vi "DataTranslation.vi"() -> (0 "DAQ Error":errorcluster)   [LabVIEW 2017]
doc: "This vi will take data with multiple DT boxes for an arbitrary number of channels either differentially or single ended, depending upon how you have wired the boxes up."
uses:
  Controls/DT_Cluster.ctl
  Controls/DT_Mode.ctl
  Globals/Meas_global.vi
  <userlib>/LV-Link3/PolySubVIs/DtOLReadMultiple2D.vi
  <userlib>/LV-Link3/PolySubVIs/DtOLTriggerDigital.vi
  <userlib>/LV-Link3/PolySubVIs/DtOLStartNormal.vi
  <userlib>/LV-Link3/PolySubVIs/DtOLTimingSetInput.vi
  <userlib>/LV-Link3/PolySubVIs/DtCreateCtrRateChan.vi
  <userlib>/LV-Link3/PolySubVIs/DtCreateAinChan.vi
  Globals/Trav_pos_global.vi
  Globals/Extra_Commands_Global.vi
  Globals/Dynamic_call_global.ph.vi
panel:
  out "Array":T1[](array[typedef])
  out "Waveform Graph":dbl[][](graph)
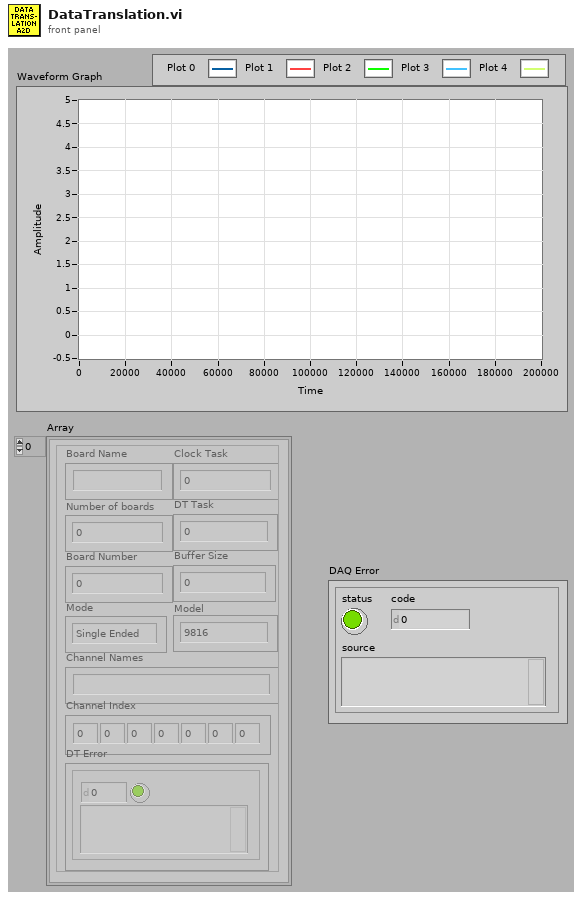
[diagram p1: front panel]
types:
  T1 = typedef "DT_Cluster.ctl" = cluster{"Board Name":string, "Number of boards":u32, "Board Number":u32, "Channel Names":string, "Channel Index":i32[], "DT Task":i32, "DT Error":errorcluster, "Mode":T2, "Buffer Size":u32, "Clock Task":i32, "Model":enum16{"9816", "9836", "9853"}}
  T2 = typedef "DT_Mode.ctl" = enum16{"Single Ended", "Differential"}
  T3 = typedef "Trigger_Mode.ctl" = enum16{"Free Running", "Start on Trigger", "Trigger Every Block", "Trigger Every Sample"}
  T4 = typedef "LDA_Setup.ctl" = cluster{"dimensions":enum16{"1D", "2D"}, "Analogue Freq Multiplier":dbl}
  T5 = enum32{"Internal Clock", "External Clock", "No Timing"}
  T6 = typedef "Traverse_cluster.ctl" = cluster{"Start X":sgl, "Start Y":sgl, "Start Z":sgl, "End X":sgl, "End Y":sgl, "End Z":sgl, "No. of pts.":i32, "Spacing":T7, "Filename":path, "Tunnel Speed":dbl, "Averaging time (min)":dbl, "Extra Commands":string, "Carrier_1 Q (l/min)":dbl, "Carrier_2 Q (l/min)":dbl, "Trace Gas Concentration (%)":dbl, "Specific Arguments":string, "Comments":string, "Row No":i32, "Row Type Selector":T8, "Completion time":string, "Row Duration (mins)":dbl, "No. of Valid pts.":i32, "Meas Setup File":string}
  T7 = typedef "Spacing.ctl" = enum16{"Linear", "Log", "Gauss", "Specified", "N/A"}
  T8 = typedef "Multi_run_mode.ctl" = enum16{"Move Traverse Only", "Set Tunnel Speed Only", "Set Source Only", "Set Measurement Conditions", "Single Measurement", "Vertical Profile", "Lateral Profile", "Longitudinal Profile", "Explore Volume", "Multi-Axis Profile", "Auto Calibrate", "Meas Fast FID Bkgnd", "Check Beam Power", "Scanning Valve Measurement", "Run VI Named:", "Set ADAM Ch", "Wait (minutes)", "Send Message", "Synchronize With:", "Fall Back to this Row", "Turn Off Row Repeating", "Blank Row", "Traverse 3D Volume"}
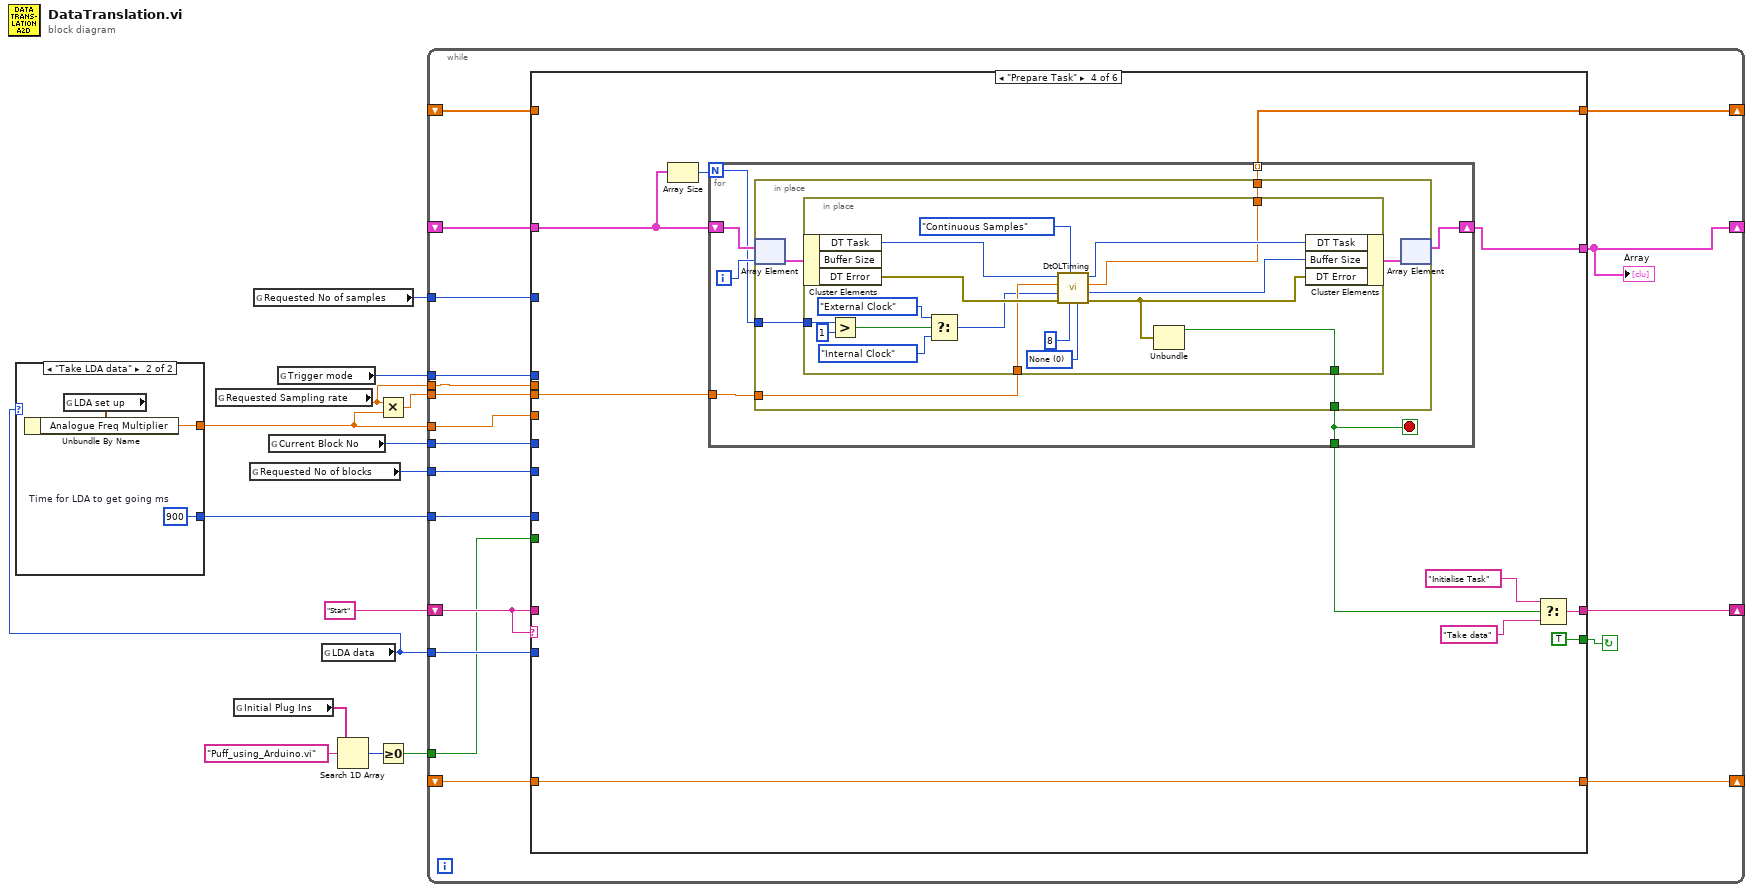
[diagram p0: block diagram]
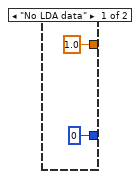
[diagram p2: hidden frame]
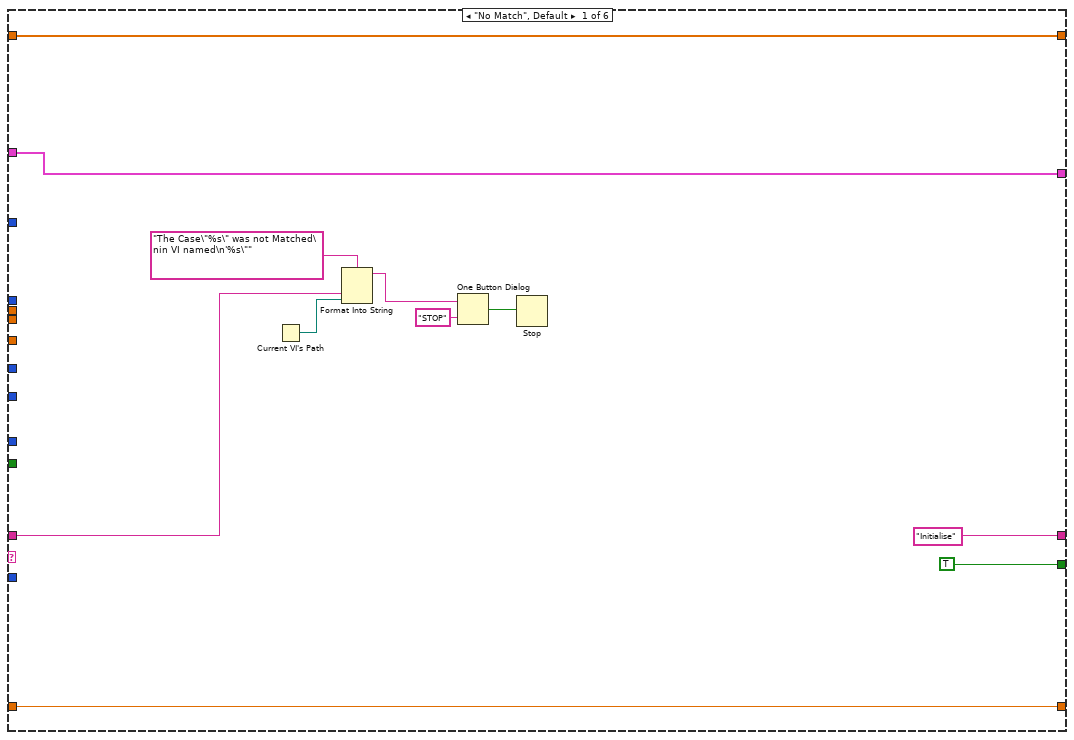
[diagram p3: hidden frame]
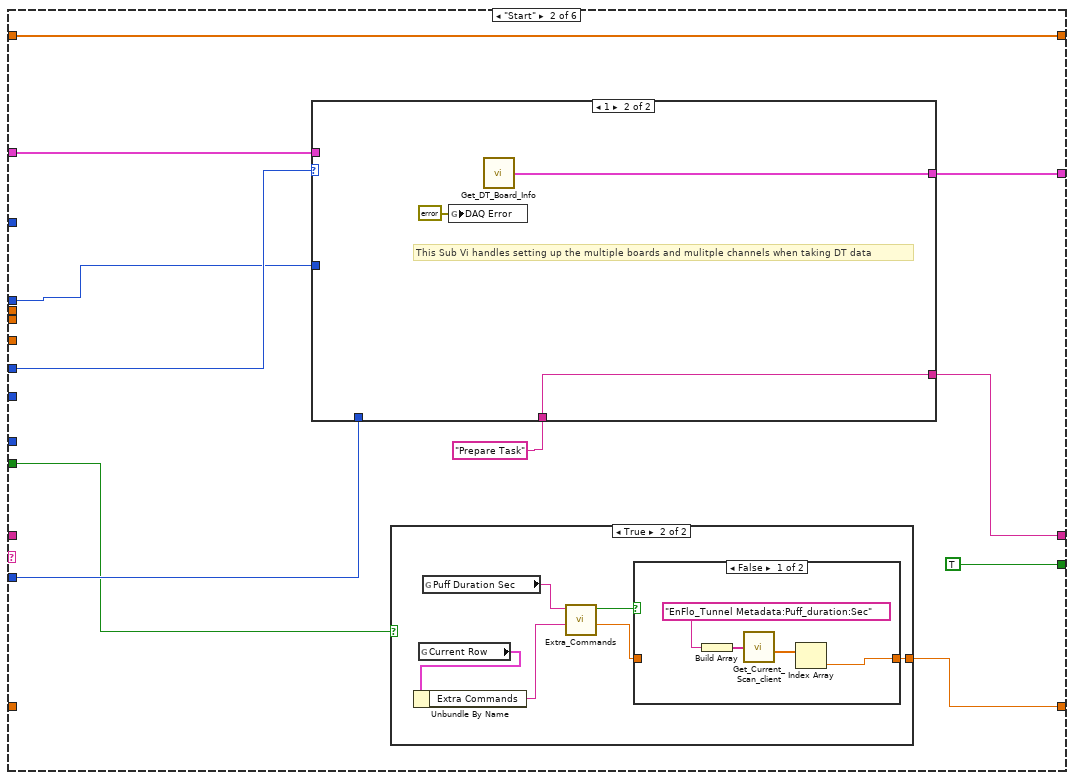
[diagram p4: hidden frame]
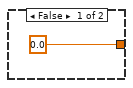
[diagram p5: hidden frame]
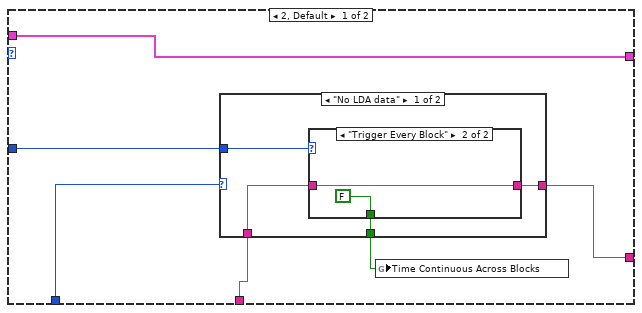
[diagram p7: hidden frame]
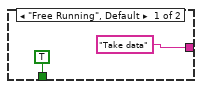
[diagram p8: hidden frame]
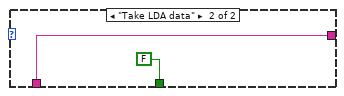
[diagram p9: hidden frame]
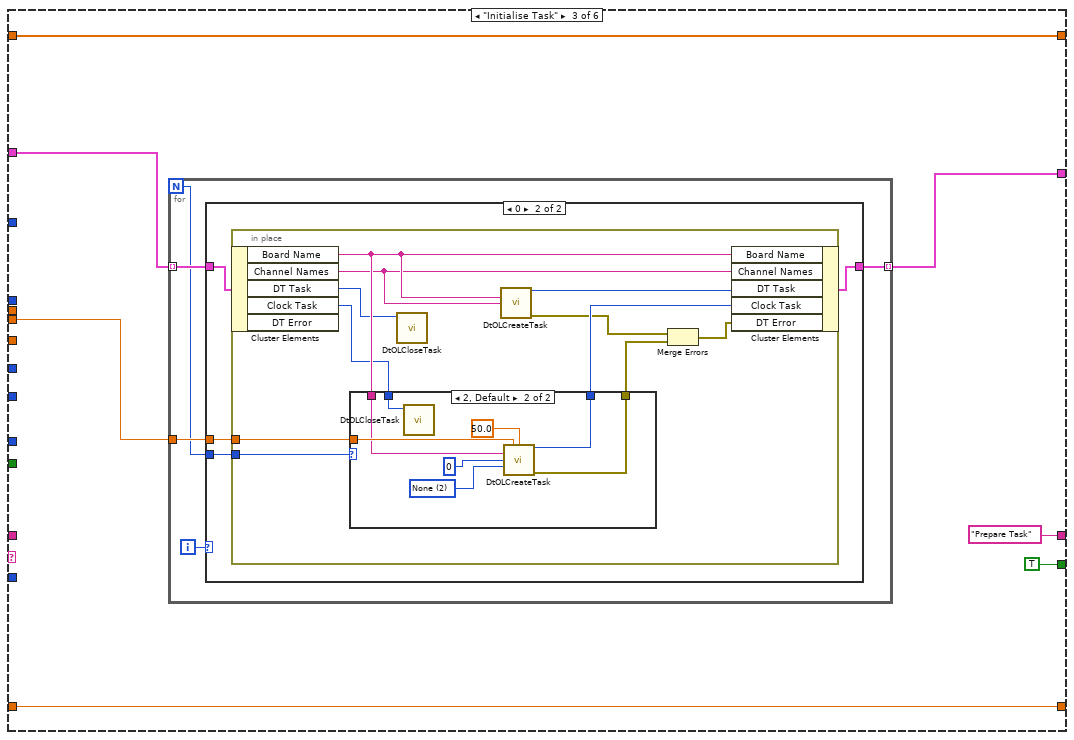
[diagram p10: hidden frame]
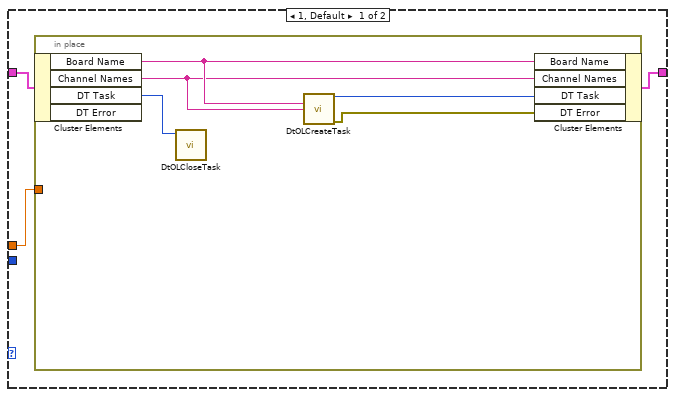
[diagram p11: hidden frame]
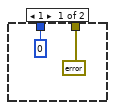
[diagram p12: hidden frame]
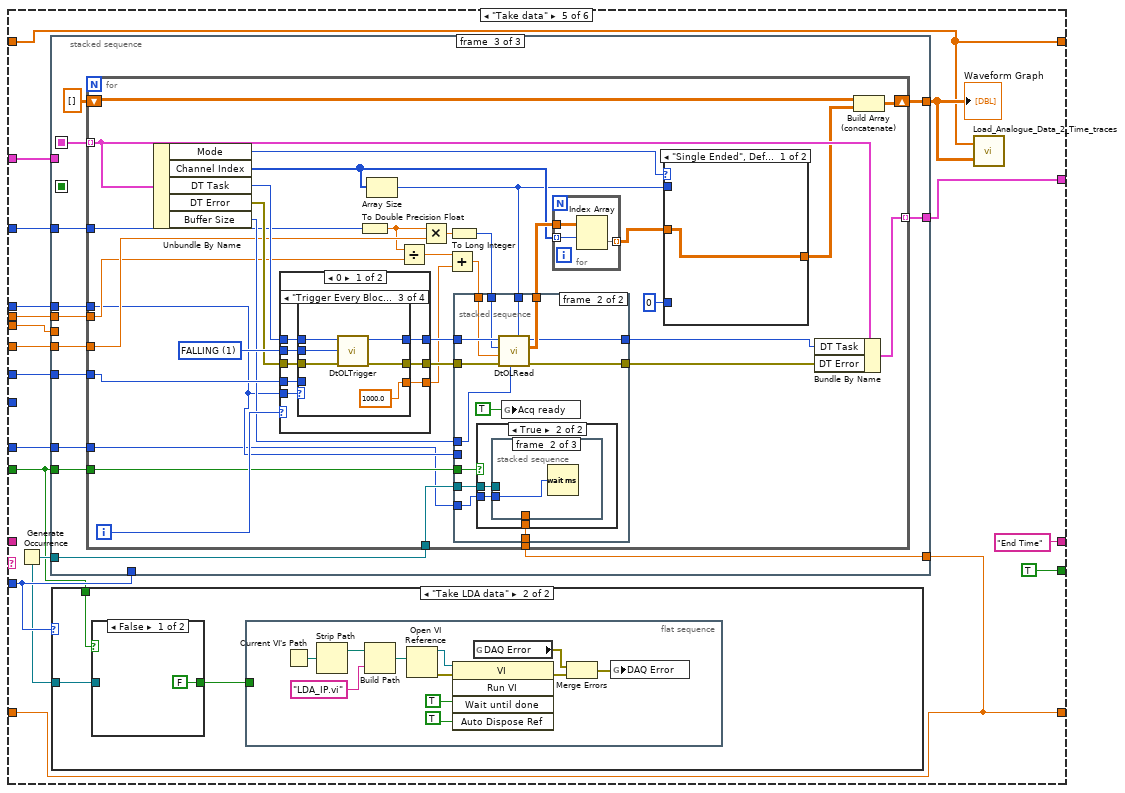
[diagram p13: hidden frame]
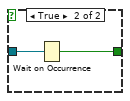
[diagram p15: hidden frame]
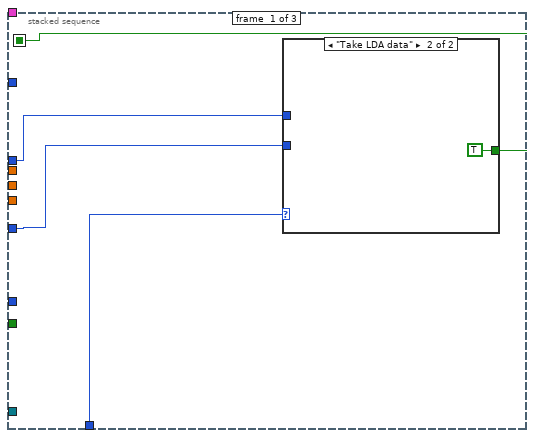
[diagram p16: hidden frame]
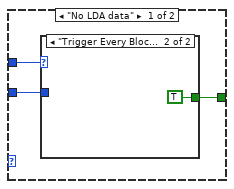
[diagram p17: hidden frame]
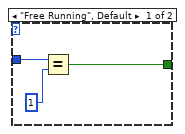
[diagram p18: hidden frame]
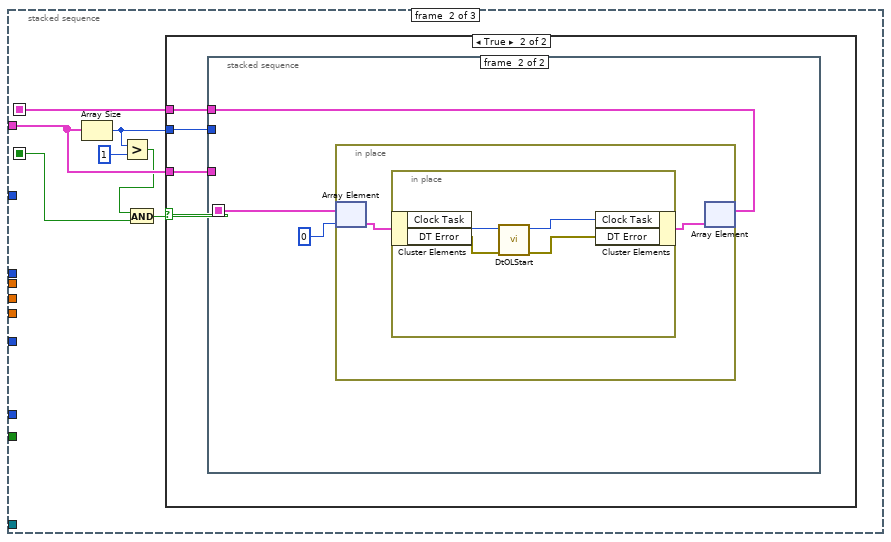
[diagram p19: hidden frame]
diagram:
  n1 = global read "Meas_global.vi" "Requested Sampling rate"() -> (w9:dbl)
  n2 = global read "Dynamic_call_global.ph.vi" "Initial Plug Ins"() -> (w5:string[])
  n3 = global read "Meas_global.vi" "Requested No of blocks"() -> (w8:i32)
  n4 = global read "Meas_global.vi" "Requested No of samples"() -> (w13:i32)
  n5 = global read "Meas_global.vi" "Current Block No"() -> (w11:i32)
  n6 = global read "Meas_global.vi" "Trigger mode"() -> (w12:T3)
  n7 = global read "Meas_global.vi" "LDA data"() -> (w6:enum16{"No LDA data", "Take LDA data"})
  n8 = case shown="\"Take LDA data\"" w6 {
    tunnel: [1.0 ("Analogue Freq Multiplier") w18] -> w7
    tunnel: [u32 0 ("Time for LDA to get going ms") w17] -> w1
    frame "No LDA data" {
    }
    frame "Take LDA data" {
      w17 = u32 900  # Time for LDA to get going ms
      n9 = global read "Meas_global.vi" "LDA set up"() -> (w19:T4)
      n10 = Unbundle By Name(w19) -> ("Analogue Freq Multiplier"=w18:dbl)
    }
  }
  n11 = Search 1D Array(1D array=w5, element="Puff_using_Arduino.vi") -> (index of element=w3:i32)  [unwired: 1 in]
  n12 = Multiply(x=w9, y=w7) -> (x*y=w10:dbl)
  n13 = Greater Or Equal To 0?(x=w3) -> (x >= 0?=w2:bool)
  n14 = while {
    shift-left: "Start" -> [w37]
    shift-right: [w38] -> _
    tunnel: w10 -> [w36]
    tunnel: w13 -> [w35]
    tunnel: w11 -> [w34]
    tunnel: w12 -> [w32]
    shift-right: [w31] -> _
    shift-left: _ -> [w30]
    tunnel: w6 -> [w29]
    tunnel: w7 -> [w28]
    tunnel: w9 -> [w27]
    tunnel: w8 -> [w26]
    tunnel: w2 -> [w25]
    shift-right: [w24] -> _
    shift-left: _ -> [w23]
    tunnel: w1 -> [w22]
    shift-right: [w21] -> _
    shift-left: _ -> [w20]
    stop <- w33 continue-if-true
    n15 = case shown="\"Prepare Task\"" w37 {
      tunnel: ["Initialise" w56 "Prepare Task" w144 "End Time" "" ("f")] -> w38
      tunnel: w37 -> [w45 _ _ _ _ _]
      tunnel: w36 -> [_ _ w96 w140 w185 _]
      tunnel: w35 -> [_ _ _ _ w193 _]
      tunnel: w34 -> [_ w57 _ _ w191 w386]
      tunnel: [TRUE TRUE TRUE TRUE TRUE FALSE] -> w33
      tunnel: w32 -> [_ w53 _ _ w190 _]
      tunnel: w30 -> [w41 w58 w94 w139 w189 w390]
      tunnel: [w41 w59 w95 w141 w188 w389] -> w31
      tunnel: w29 -> [_ w54 _ _ w184 _]
      tunnel: w28 -> [_ _ _ _ w187 _]
      tunnel: w27 -> [_ _ _ _ w186 _]
      tunnel: w26 -> [_ _ _ _ _ w387]
      tunnel: w25 -> [_ w52 _ _ w181 _]
      tunnel: [w40 w51 w93 w138 w182 w382] -> w24
      tunnel: w23 -> [w40 _ w93 w138 w182 w382]
      tunnel: w22 -> [_ _ _ _ w180 _]
      tunnel: [w39 w50 w92 w137 w178 w381] -> w21
      tunnel: w20 -> [w39 w50 w92 _ w178 w381]
      frame "No Match", Default {
        n16 = Current VI's Path() -> (path=w44:path)
        n17 = Format Into String(format string="The Case\"%s\" was not Matched\nin VI named\n'%s\"" ("Format String"), w45, w44) -> (resulting string=w48:string)  [unwired: 2 in, 1 out]
        n18 = One Button Dialog(message=w48, button name ("OK")="STOP") -> (true=w46:bool)
        n19 = Stop(stop? (T)=w46) -> ()
      }
      frame "Start" {
        n20 = case shown="1" w57 {
          tunnel: [w78 w91] -> w59
          tunnel: w58 -> [w78 _]
          tunnel: [w76 w89] -> w56
          tunnel: "Prepare Task" -> [w75 w89]
          tunnel: w54 -> [w77 _]
          tunnel: w53 -> [w74 _]
          frame 2, Default {
            n21 = case shown="\"No LDA data\"" w77 {
              tunnel: [w82 w88] -> w76
              tunnel: w75 -> [w80 w88]
              tunnel: w74 -> [w81 _]
              tunnel: [w79 FALSE ("Time Continuous across Blocks")] -> w73
              frame "No LDA data" {
                n22 = case shown="\"Trigger Every Block\"" w81 {
                  tunnel: ["Take data" w86] -> w82
                  tunnel: w80 -> [_ w86]
                  tunnel: [TRUE ("Time Continuous across Blocks") FALSE ("Time Continuous across Blocks")] -> w79
                  frame "Free Running", Default {
                  }
                  frame "Trigger Every Block" {
                  }
                }
              }
              frame "Take LDA data" {
              }
            }
            n23 = global write "Meas_global.vi" "Time Continuous Across Blocks"(w73) -> ()
          }
          frame 1 {
            # "This Sub Vi handles setting up the multiple boards and mulitple channels when taking DT data"
            n24 = global write "Meas_global.vi" "DAQ Error"(errorcluster {"status"=FALSE, "code"=0, "source"=""} ("DAQ Error")) -> ()
            n25 = call "Get_DT_Board_Info.vi"() -> ("DT Cluster Array"=w91:T1[])  [unwired: 5 in]
          }
        }
        n26 = case shown="True" w52 {
          tunnel: [0.0 w67] -> w51
          frame False {
          }
          frame True {
            n27 = global read "Trav_pos_global.vi" "Current Row"() -> (w66:T6)
            n28 = Unbundle By Name(w66) -> ("Extra Commands"=w65:string)
            n29 = global read "Extra_Commands_Global.vi" "Puff Duration Sec"() -> (w64:string)
            n30 = call "Extra_Commands.vi"("String to Search"=w65, "Command"=w64) -> ("Numeric Value"=w62:dbl, "Command Found"=w63:bool)  [unwired: 2 in, 2 out]
            n31 = case shown="False" w63 {
              tunnel: [w68 w72] -> w67
              tunnel: w62 -> [_ w72]
              frame False {
                n32 = Build Array("EnFlo_Tunnel Metadata:Puff_duration:Sec") -> (w70:string[])
                n33 = call "Get_Current_Scan_client.vi"("ADAM Ch Names"=w70) -> ("Numerical Values"=w71:dbl[])  [unwired: 1 in, 2 out]
                n34 = Index Array(array=w71) -> (element=w68:dbl)  [unwired: 1 in]
              }
              frame True {
              }
            }
          }
        }
      }
      frame "Initialise Task" {
        n35 = for {
          N -> [w99]
          tunnel: w94 -> [w103] mode=indexing
          tunnel: w96 -> [w102]
          tunnel: [w101] -> w95 mode=indexing
          i -> [w100]
          n36 = case shown="0" w100 {
            tunnel: w103 -> [w106 w115]
            tunnel: w102 -> [w105 w114]
            tunnel: [w104 w113] -> w101
            tunnel: w99 -> [_ w112]
            frame 1, Default {
              n37 = in-place {
                in-place-border: w105 -> [_]
                n38 = in-place-cluster #1(w106) -> ("Board Name"=w111:string, "Channel Names"=w108:string, "DT Task"=w107:i32)  [unwired: 1 out]
                n39 = call <userlib>:"DtOLCloseTask.vi"("Task in"=w107) -> ()  [unwired: 10 in, 1 out]
                n40 = call-poly <userlib>:"DtOLCreateTask.vi"("Board Name"=w111, "Channel"=w108) -> ("Task out"=w110:i32, "error out"=w109:errorcluster)  [unwired: 11 in, 1 out]
                n41 = in-place-cluster #1("Board Name"=w111, "Channel Names"=w108, "DT Task"=w110, "DT Error"=w109) -> (w104:T1)
              }
            }
            frame 0 {
              n42 = in-place {
                in-place-border: w114 -> [w126]
                in-place-border: w112 -> [w117]
                n43 = in-place-cluster #2(w115) -> ("Board Name"=w124:string, "Channel Names"=w119:string, "DT Task"=w118:i32, "Clock Task"=w116:i32)  [unwired: 1 out]
                n44 = case shown="2, Default" w117 {
                  tunnel: w126 -> [_ w133]
                  tunnel: [errorcluster {"status"=FALSE, "code"=0, "source"=""} ("error out") w132] -> w125
                  tunnel: w124 -> [_ w131]
                  tunnel: [0 ("Task out") w130] -> w122
                  tunnel: w116 -> [_ w129]
                  frame 1 {
                  }
                  frame 2, Default {
                    w136 = 2 items=["LowLevel", "HighLevel", "None"] ("Gate Type")
                    n45 = call <userlib>:"DtOLCloseTask.vi"("Task in"=w129) -> ()  [unwired: 10 in, 1 out]
                    n46 = call-poly <userlib>:"DtOLCreateTask.vi"("Requested\nFrequency (Hz)"=w133, "Duty Cycle"=50.0, "Board Name"=w131, "Counter Num"=u32 0, "Gate Type"=w136) -> ("Task out"=w130:i32, "error out"=w132:errorcluster)  [unwired: 8 in, 1 out]
                  }
                }
                n47 = call <userlib>:"DtOLCloseTask.vi"("Task in"=w118) -> ()  [unwired: 10 in, 1 out]
                n48 = call-poly <userlib>:"DtOLCreateTask.vi"("Board Name"=w124, "Channel"=w119) -> ("Task out"=w123:i32, "error out"=w121:errorcluster)  [unwired: 11 in, 1 out]
                n49 = Merge Errors(w121, w125) -> (w120:errorcluster)
                n50 = in-place-cluster #2("Board Name"=w124, "Channel Names"=w119, "DT Task"=w123, "Clock Task"=w122, "DT Error"=w120) -> (w113:T1)
              }
            }
          }
        }
      }
      frame "Prepare Task" {
        n51 = Array Size(array=w139) -> (size(s)=w143:i32)
        n52 = for {
          N: w143 -> [w149]
          shift-right: [w151] -> w141
          shift-left: w139 -> [w153]
          tunnel: [w154] -> w142
          tunnel: w140 -> [w150]
          tunnel: [w148] -> w137 mode=indexing
          i -> [w152]
          stop <- w154 stop-if-true
          n53 = in-place {
            in-place-border: [w160] -> w154
            in-place-border: w150 -> [w157]
            in-place-border: w149 -> [w156]
            in-place-border: [w155] -> w148
            n54 = in-place-array #3(w153, w152) -> (w159:T1)
            n55 = in-place {
              in-place-border: [w172] -> w160
              in-place-border: w157 -> [w171]
              in-place-border: w156 -> [w170]
              in-place-border: [w161] -> w155
              w163 = 0 items=["None", "Master", "Slave"] ("Sync Mode")
              n56 = in-place-cluster #4(w159) -> ("DT Task"=w177:i32, "DT Error"=w176:errorcluster)  [unwired: 1 out]
              n57 = Greater?(x=w170, y=1) -> (0:w168:bool)
              n58 = Select(t=T5."External Clock" ("Timing"), s=w168, f=T5."Internal Clock" ("Timing")) -> (s? t:f=w165:T5)
              n59 = call-poly <userlib>:"DtOLTiming.vi"("Sync Mode"=w163, "Num Buffers"=u32 8, "Sample Mode"=enum16{"Finite Samples", "Continuous Samples"}."Continuous Samples", "error in (no error)"=w176, "Timing"=w165, "Sample Freq (Hz)"=w171, "Task in"=w177) -> ("error out"=w173:errorcluster, "Buffer Size"=w175:u32, "Actual Sample Freq"=w161:dbl, "Task out"=w174:i32)  [unwired: 1 in]
              n60 = Unbundle(w173) -> ("status"=w172:bool)  [unwired: 2 out]
              n61 = in-place-cluster #4("DT Task"=w174, "Buffer Size"=w175, "DT Error"=w173) -> (w158:T1)
            }
            n62 = in-place-array #3(w158) -> (w151:T1[])  [unwired: 1 out]
          }
        }
        n63 = Select(t="Initialise Task", s=w142, f="Take data") -> (s? t:f=w144:string)
      }
      frame "Take data" {
        n64 = Generate Occurrence() -> (w183:refnum<k4>)
        n65 = stacked-sequence {
          seq-local: [_ w230 _] -> [_ _ w260]
          seq-local: [w213 _ _] -> [_ w225 _]
          tunnel: w193 -> [_ _ w268]
          tunnel: w191 -> [w214 _ w267]
          tunnel: w190 -> [w212 _ w266]
          tunnel: w189 -> [_ w229 _]
          tunnel: [_ _ w265] -> w188
          tunnel: [_ _ w263] -> w179
          tunnel: w187 -> [_ _ w262]
          tunnel: w186 -> [_ _ w261]
          tunnel: w184 -> [w215 _ _]
          tunnel: w185 -> [_ _ _]
          tunnel: w183 -> [_ _ w259]
          tunnel: w181 -> [_ _ w258]
          tunnel: w182 -> [_ _ w257]
          tunnel: w180 -> [_ _ w256]
          frame #0 {
            n66 = case shown="\"Take LDA data\"" w215 {
              tunnel: w214 -> [w218 _]
              tunnel: [w217 TRUE] -> w213
              tunnel: w212 -> [w216 _]
              frame "No LDA data" {
                n67 = case shown="\"Trigger Every Block\"" w216 {
                  tunnel: w218 -> [w221 _]
                  tunnel: [w219 TRUE] -> w217
                  frame "Free Running", Default {
                    n68 = Equal?(x=w221, y=1) -> (x = y?=w219:bool)
                  }
                  frame "Trigger Every Block" {
                  }
                }
              }
              frame "Take LDA data" {
              }
            }
          }
          frame #1 {
            n69 = Array Size(array=w229) -> (size(s)=w228:i32)
            n70 = Greater?(x=w228, y=1) -> (0:w226:bool)
            n71 = And(x=w226, y=w225) -> (x .and. y?=w224:bool)
            n72 = case shown="True" w224 {
              tunnel: [w231 w234] -> w230
              tunnel: w229 -> [w231 w233]
              tunnel: w228 -> [_ w232]
              frame False {
              }
              frame True {
                n73 = stacked-sequence {
                  seq-local: [w235 _] -> [_ w248]
                  tunnel: [_ w247] -> w234
                  tunnel: w233 -> [w237 _]
                  tunnel: w232 -> [w236 _]
                  frame #0 {
                    n74 = for {
                      N: w236 -> [_]
                      shift-right: [w238] -> w235
                      shift-left: w237 -> [w239]
                      i -> [w240]
                      n75 = in-place {
                        n76 = in-place-array #5(w239, w240) -> (w242:T1)
                        n77 = in-place {
                          n78 = in-place-cluster #6(w242) -> ("DT Task"=w246:i32, "DT Error"=w245:errorcluster)
                          n79 = call-poly <userlib>:"DtOLStart.vi"("error in (no error)"=w245, "Task in"=w246) -> ("error out"=w244:errorcluster, "Task out"=w243:i32)  [unwired: 8 in]
                          n80 = in-place-cluster #6("DT Task"=w243, "DT Error"=w244) -> (w241:T1)
                        }
                        n81 = in-place-array #5(w241) -> (w238:T1[])  [unwired: 1 out]
                      }
                    }
                  }
                  frame #1 {
                    n82 = in-place {
                      n83 = in-place-array #7(w248, 0) -> (w251:T1)
                      n84 = in-place {
                        n85 = in-place-cluster #8(w251) -> ("Clock Task"=w254:i32, "DT Error"=w255:errorcluster)
                        n86 = call-poly <userlib>:"DtOLStart.vi"("error in (no error)"=w255, "Task in"=w254) -> ("error out"=w252:errorcluster, "Task out"=w253:i32)  [unwired: 8 in]
                        n87 = in-place-cluster #8("Clock Task"=w253, "DT Error"=w252) -> (w250:T1)
                      }
                      n88 = in-place-array #7(w250) -> (w247:T1[])  [unwired: 1 out]
                    }
                  }
                }
              }
            }
          }
          frame #2 {
            n89 = for {
              tunnel: w268 -> [w283]
              tunnel: w267 -> [w301]
              tunnel: w266 -> [w270]
              tunnel: w260 -> [w297] mode=indexing
              tunnel: [w296] -> w265 mode=indexing
              shift-right: [w293] -> w263
              shift-left: dbl[][] [] -> [w292]
              tunnel: w262 -> [w282]
              tunnel: w261 -> [w280]
              tunnel: w259 -> [w273]
              tunnel: w258 -> [w272]
              tunnel: w257 -> [w271]
              tunnel: w256 -> [w269]
              i -> [w290]
              w302 = 1 items=["RISING", "FALLING"] ("External Trigger Polarity")
              n90 = Unbundle By Name(w297) -> ("Mode"=w287:T2, "Channel Index"=w294:i32[], "DT Task"=w300:i32, "DT Error"=w299:errorcluster, "Buffer Size"=w285:u32)
              n91 = case shown="0" w290 {
                tunnel: [w346 w377] -> w303
                tunnel: w302 -> [w345 _]
                tunnel: w301 -> [w344 _]
                tunnel: w270 -> [w343 _]
                tunnel: w300 -> [w342 w377]
                tunnel: w299 -> [w341 w376]
                tunnel: [w340 w376] -> w298
                tunnel: [w339 10.0 ("x")] -> w277
                frame 0 {
                  n92 = case shown="\"Trigger Every Block\"" w343 {
                    tunnel: [w349 w354 w369 w374] -> w346
                    tunnel: w342 -> [w349 w355 w371 w374]
                    tunnel: w344 -> [_ w356 _ _]
                    tunnel: w345 -> [_ w353 w370 _]
                    tunnel: w341 -> [w348 w352 w368 w373]
                    tunnel: [w348 w351 w367 w373] -> w340
                    tunnel: [10.0 ("x") w350 1000.0 ("x") 1000.0 ("x")] -> w339
                    frame "Free Running" {
                    }
                    frame "Start on Trigger" {
                      n93 = case shown="1" w356 {
                        tunnel: w355 -> [w362 w365]
                        tunnel: w352 -> [w361 w364]
                        tunnel: [w359 w365] -> w354
                        tunnel: [w360 w364] -> w351
                        tunnel: w353 -> [w358 _]
                        tunnel: [1000.0 ("x") 10.0 ("x")] -> w350
                        frame 1 {
                          n94 = call-poly <userlib>:"DtOLTrigger.vi"("error in (no error)"=w361, "External Trigger Polarity"=w358, "Task in"=w362) -> ("error out"=w360:errorcluster, "Task out"=w359:i32)  [unwired: 7 in]
                        }
                        frame 2, Default {
                        }
                      }
                    }
                    frame "Trigger Every Block" {
                      n95 = call-poly <userlib>:"DtOLTrigger.vi"("error in (no error)"=w368, "External Trigger Polarity"=w370, "Task in"=w371) -> ("error out"=w367:errorcluster, "Task out"=w369:i32)  [unwired: 7 in]
                    }
                    frame "Trigger Every Sample" {
                    }
                  }
                }
                frame 1, Default {
                }
              }
              n96 = To Double Precision Float(number=w283) -> (double precision float=w275:dbl)
              n97 = Array Size(array=w294) -> (size(s)=w276:i32)
              n98 = Divide(x=w275, y=w280) -> (x/y=w278:dbl)
              n99 = Multiply(x=w275, y=w282) -> (x*y=w281:dbl)
              n100 = Add(x=w278, y=w277) -> (x+y=w291:dbl)
              n101 = To Long Integer(number=w281) -> (32bit integer=w274:i32)
              n102 = stacked-sequence {
                tunnel: w303 -> [_ w320]
                tunnel: w298 -> [_ w319]
                tunnel: [_ w318] -> w295
                tunnel: w291 -> [_ w317]
                tunnel: [_ w316] -> w289
                tunnel: w285 -> [_ w312]
                tunnel: [_ w315] -> w284
                tunnel: w274 -> [_ w314]
                tunnel: w276 -> [_ w313]
                tunnel: w273 -> [_ w310]
                tunnel: w272 -> [_ w309]
                tunnel: w271 -> [_ w308]
                tunnel: w270 -> [w305 _]
                tunnel: w269 -> [w304 w307]
                frame #0 {
                  n103 = case shown="\"Free Running\"" w305 {
                    tunnel: w304 -> [w306 _]
                    frame "Free Running" {
                      n104 = Wait (ms)(milliseconds to wait=w306) -> ()  [unwired: 1 out]
                    }
                    frame Default {
                    }
                  }
                }
                frame #1 {
                  n105 = case shown="True" w309 {
                    tunnel: w310 -> [_ w323]
                    tunnel: w308 -> [_ w322]
                    tunnel: w307 -> [_ w321]
                    frame False {
                    }
                    frame True {
                      n106 = stacked-sequence {
                        tunnel: w323 -> [w324 _ _]
                        tunnel: w322 -> [_ _ w326]
                        tunnel: w321 -> [_ w325 _]
                        frame #0 {
                          n107 = Set Occurrence(w324) -> ()
                        }
                        frame #1 {
                          n108 = Wait (ms)(milliseconds to wait=w325) -> ()  [unwired: 1 out]
                        }
                        frame #2 {
                          n109 = call "Puff_using_Arduino_oneshot.vi"("Puff_duration:Sec"=w326) -> ()  [unwired: 7 in]
                        }
                      }
                    }
                  }
                  n110 = call-poly <userlib>:"DtOLRead.vi"("Number Chan to Read"=w313, "Buffer size"=w312, "error in (no error)"=w319, "Timeout"=w317, "Samples Per Channel"=w314, "Task in"=w320) -> ("error out"=w315:errorcluster, "2D Data out"=w318:dbl[][], "Task out"=w316:i32)  [unwired: 1 in, 2 out]
                  n111 = global write "Meas_global.vi" "Acq ready"(TRUE ("Acq ready")) -> ()
                }
              }
              n112 = for {
                tunnel: w294 -> [w380] mode=indexing
                tunnel: w295 -> [w379]
                tunnel: [w378] -> w279 mode=indexing
                n113 = Index Array(array=w379, index (row)=w380) -> (element=w378:dbl[])  [unwired: 1 in]
              }
              n114 = case shown="\"Single Ended\", Default" w287 {
                tunnel: w279 -> [w327 w332]
                tunnel: [w327 w331] -> w288
                tunnel: 0 ("size(s)") -> [_ w330]
                tunnel: w276 -> [_ w329]
                frame "Single Ended", Default {
                }
                frame "Differential" {
                  n115 = expression code="0.5*x"(w329) -> (w328:i32)
                  n116 = for {
                    N: w328 -> [_]
                    tunnel: w332 -> [w338]
                    shift-right: [w337] -> _
                    shift-left: w330 -> [w336]
                    tunnel: [w334] -> w331 mode=indexing
                    n117 = Index Array(array=w338, index (row) #1=w336) -> (element #1=w333:dbl[], element #2=w335:dbl[])  [unwired: 3 in]
                    n118 = expression code="x+2"(w336) -> (w337:i32)
                    n119 = Subtract(x=w333, y=w335) -> (x-y=w334:dbl[])
                  }
                }
              }
              n120 = Bundle By Name(cluster=w297, "DT Task"=w289, "DT Error"=w284) -> (w296:T1)
              n121 = Build Array (concatenate)(w292, w288) -> (w293:dbl[][])
            }
          }
        }
        "Waveform Graph" <- w179
        n122 = case shown="\"Take LDA data\"" w184 {
          tunnel: w183 -> [_ w197]
          tunnel: w181 -> [_ w195]
          frame "No LDA data", Default {
          }
          frame "Take LDA data" {
            n123 = case shown="False" w195 {
              tunnel: w197 -> [_ w200]
              tunnel: [FALSE ("timed out") w199] -> w196
              frame False {
              }
              frame True {
                n124 = Wait on Occurrence(2:w200) -> (0:w199:bool)  [unwired: 2 in]
              }
            }
            n125 = flat-sequence {
              tunnel: w196 -> [_]
              frame #0 {
                n126 = Current VI's Path() -> (path=w205:path)
                n127 = Strip Path(path=w205) -> (stripped path=w201:path)  [unwired: 1 out]
                n128 = Build Path(base path=w201, name or relative path="LDA_IP.vi") -> (appended path=w206:path)
                n129 = Open VI Reference(vi path=w206) -> (vi reference=w209:refnum<vi>, error out=w210:errorcluster)  [unwired: 5 in]
                n130 = invoke class="VI" method="Run VI"(reference=w209, error in=w210, "Wait until done"=TRUE ("Wait Until Done"), "Auto Dispose Ref"=TRUE ("Wait until done")) -> (error out=w203:errorcluster)  [unwired: 1 in, 4 out]
                n131 = global read "Meas_global.vi" "DAQ Error"() -> (w204:errorcluster)
                n132 = Merge Errors(w204, w203) -> (w202:errorcluster)
                n133 = global write "Meas_global.vi" "DAQ Error"(w202) -> ()
              }
            }
          }
        }
        n134 = call "Load_Analogue_Data_2_Time_traces.vi"("Voltage Array"=w179, "Sampling Rate (Hz)"=w178) -> ()  [unwired: 1 in]
      }
      frame "End Time" {
        n135 = Equal?(x=w386, y=w387) -> (x = y?=w384:bool)
        n136 = case shown="True" w384 {
          tunnel: w390 -> [w393 w395]
          tunnel: [w393 w394] -> w389
          frame False {
          }
          frame True {
            n137 = for {
              N -> [w396]
              tunnel: w395 -> [w399] mode=indexing
              tunnel: [w398] -> w394 mode=indexing
              i -> [w397]
              n138 = case shown="0" w397 {
                tunnel: w399 -> [w401 w408]
                tunnel: [w400 w407] -> w398
                tunnel: w396 -> [_ w406]
                frame 1, Default {
                  n139 = in-place {
                    n140 = in-place-cluster #9(w401) -> ("DT Task"=w405:i32, "DT Error"=w404:errorcluster)
                    n141 = call <userlib>:"DtOLCloseTask.vi"("Error in"=w404, "Task in"=w405) -> ("Error Out"=w403:errorcluster)  [unwired: 9 in]
                    n142 = in-place-cluster #9("DT Task"=0, "DT Error"=w403) -> (w400:T1)
                  }
                }
                frame 0 {
                  n143 = in-place {
                    in-place-border: w406 -> [w409]
                    n144 = in-place-cluster #10(w408) -> ("DT Task"=w415:i32, "DT Error"=w414:errorcluster, "Clock Task"=w412:i32)
                    n145 = case shown="2, Default" w409 {
                      tunnel: [errorcluster {"status"=FALSE, "code"=0, "source"=""} ("Error Out") w420] -> w417
                      tunnel: w412 -> [_ w419]
                      frame 1 {
                      }
                      frame 2, Default {
                        n146 = call <userlib>:"DtOLCloseTask.vi"("Task in"=w419) -> ("Error Out"=w420:errorcluster)  [unwired: 10 in]
                      }
                    }
                    n147 = call <userlib>:"DtOLCloseTask.vi"("Error in"=w414, "Task in"=w415) -> ("Error Out"=w413:errorcluster)  [unwired: 9 in]
                    n148 = Merge Errors(w413, w417) -> (w416:errorcluster)
                    n149 = in-place-cluster #10("DT Task"=0, "DT Error"=w416, "Clock Task"=0) -> (w407:T1)
                  }
                }
              }
            }
          }
        }
        n150 = global write "Meas_global.vi" "Acq ready"(FALSE ("Acq ready")) -> ()
        n151 = global read "Meas_global.vi" "DAQ Error"() -> (w385:errorcluster)
        n152 = for {
          tunnel: w389 -> [w424] mode=indexing
          shift-right: [w421] -> w388
          shift-left: w385 -> [w422]
          n153 = Unbundle By Name(w424) -> ("DT Error"=w423:errorcluster)
          n154 = Merge Errors(w422, w423) -> (w421:errorcluster)
        }
        "DAQ Error" <- w388
        n155 = global write "Meas_global.vi" "DAQ Error"(w388) -> ()
      }
    }
    "Array" <- w31
  }
